vi "Untitled 2 (SubVI).vi"(6 "L0":i32, 9 "L1":i32, 10 "X":i32, 11 "Y":i32) -> (7 "Numeric":dbl)   [LabVIEW 2014]
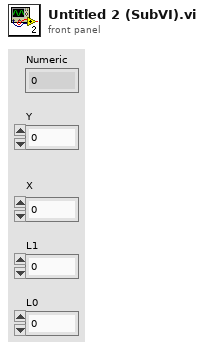
[diagram p1: front panel]
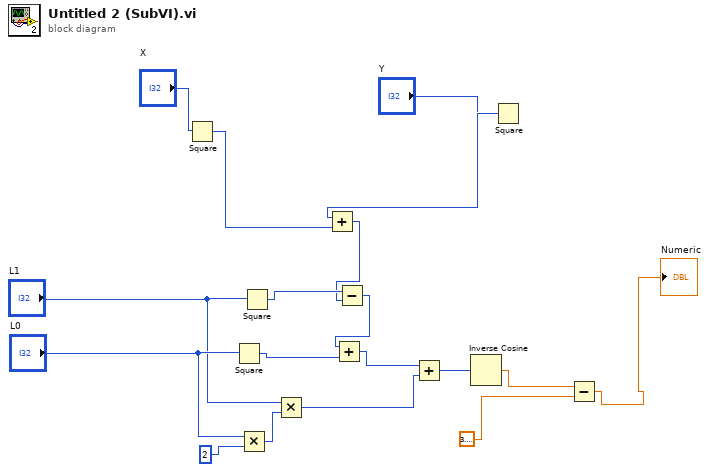
[diagram p0: block diagram]
diagram:
  n1 = Square(x="X") -> (x^2=w4:i32)
  n2 = Square(x="L0") -> (x^2=w7:i32)
  n3 = Multiply(x="L0", y=2) -> (x*y=w11:i32)
  n4 = Square(x="L1") -> (x^2=w6:i32)
  n5 = Multiply(x="L1", y=w11) -> (x*y=w14:i32)
  n6 = Square(x="Y") -> (x^2=w2:i32)
  n7 = Add(x=w2, y=w4) -> (x+y=w5:i32)
  n8 = Subtract(x=w6, y=w5) -> (x-y=w8:i32)
  n9 = Add(x=w8, y=w7) -> (x+y=w9:i32)
  n10 = Add(x=w9, y=w14) -> (x+y=w15:i32)
  n11 = Inverse Cosine(1:w15) -> (0:w16:dbl)
  n12 = Subtract(x=w16, y=3.141592653589793) -> (x-y=→"Numeric":dbl)
